vi "freqInit.vi"(1 "频率终止":dbl=30.0, 2 "频率步进":dbl=0.1, 3 "频率起始":dbl=24.0) -> (0 "频率变化次数":dbl)   [LabVIEW 2018]
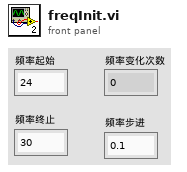
[diagram p1: front panel]
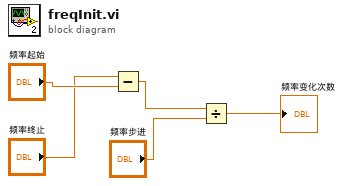
[diagram p0: block diagram]
diagram:
  n1 = Subtract(x="频率终止", y="频率起始") -> (x-y=w2:dbl)
  n2 = Divide(x=w2, y="频率步进") -> (x/y=→"频率变化次数":dbl)
